vi "Add border reading.vi"(7 "Default power":dbl, 8 "Lower border?":bool, 9 "Border frequency":dbl, 10 "Border index":i32, 11 "Power readings in":cluster{"Frequency":dbl, "Power":dbl}[](array[cluster])) -> (3 "Power readings out":cluster{"Frequency":dbl, "Power":dbl}[](array[cluster]))   [LabVIEW 2015, in "Power control.lvclass"]
uses:
  Power control.lvclass
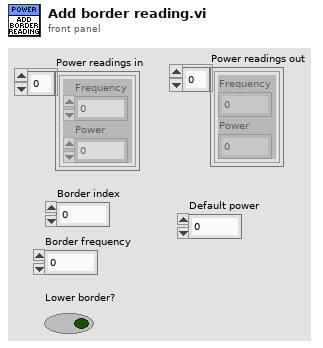
[diagram p1: front panel]
types:
  T1 = cluster{"Border frequency":dbl, "Default power":dbl}
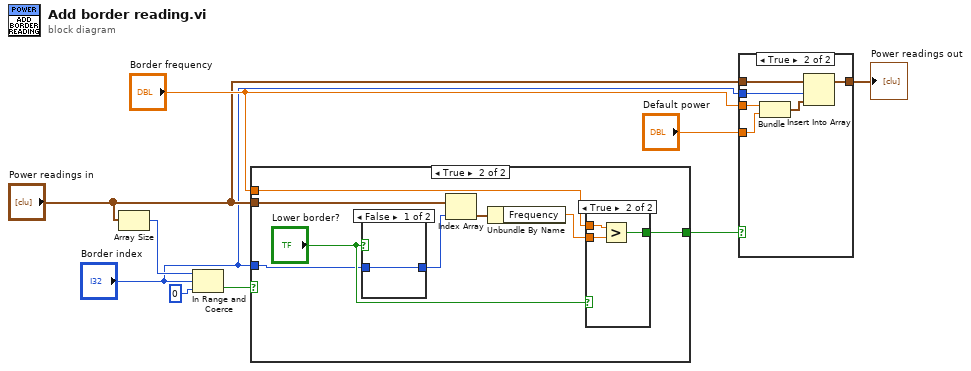
[diagram p0: block diagram]
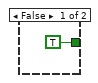
[diagram p3: hidden frame]
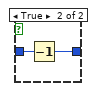
[diagram p4: hidden frame]
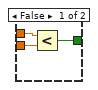
[diagram p5: hidden frame]
diagram:
  n1 = Array Size(array="Power readings in") -> (size(s)=w8:i32)
  n2 = In Range and Coerce(upper limit=w8, x="Border index", lower limit=0) -> (In Range?=w9:bool)  [unwired: 1 out]
  n3 = case shown="True" w9 {
    tunnel: "Power readings in" -> [_ w16]
    tunnel: "Border frequency" -> [_ w17]
    tunnel: [TRUE w14] -> w2
    tunnel: "Border index" -> [_ w12]
    frame False {
    }
    frame True {
      n4 = case shown="False" "Lower border?" {
        tunnel: w12 -> [w19 w21]
        tunnel: [w19 w20] -> w11
        frame False {
        }
        frame True {
          n5 = Decrement(x=w21) -> (x-1=w20:i32)
        }
      }
      n6 = Index Array(array=w16, index=w11) -> (element=w15:cluster{"Frequency":dbl, "Power":dbl})
      n7 = Unbundle By Name(w15) -> ("Frequency"=w18:dbl)
      n8 = case shown="True" "Lower border?" {
        tunnel: [w24 w27] -> w14
        tunnel: w18 -> [w22 w26]
        tunnel: w17 -> [w23 w25]
        frame False {
          n9 = Less?(x=w23, y=w22) -> (x < y?=w24:bool)
        }
        frame True {
          n10 = Greater?(x=w25, y=w26) -> (0:w27:bool)
        }
      }
    }
  }
  n11 = case shown="True" w2 {
    tunnel: "Border index" -> [_ w34]
    tunnel: "Power readings in" -> [w28 w33]
    tunnel: "Border frequency" -> [_ w31]
    tunnel: "Default power" -> [_ w30]
    tunnel: [w28 w32] -> w6
    frame False {
    }
    frame True {
      n12 = Bundle("Border frequency"=w31, "Default power"=w30) -> (w29:T1)  [unwired: 1 in]
      n13 = Insert Into Array(array=w33, index=w34, new element=w29) -> (w32:cluster{"Frequency":dbl, "Power":dbl}[])
    }
  }
  "Power readings out" <- w6
